vi "Get SMO HELP.vi"(8 "error in (no error)":errorcluster, 10 "Command":string, 11 "Inst.RP100 in":refnum<class "Inst.RP100.lvclass">) -> (0 "error out":errorcluster, 2 "output cluster":T1, 3 "Inst.RP100 out":refnum<class "Inst.RP100.lvclass">)   [LabVIEW 2019, in "Inst.RP100.lvlib" / "Inst.RP100.lvclass"]
uses:
  Inst.RP100.lvclass
  <userlib>/LevyLab/Instrument Framework/subsystems/Help/typedefs/Help--cluster.ctl
  Typedefs/setLevel--Cluster.ctl
  Typedefs/Channel--Num.ctl
  Typedefs/setState--Cluster.ctl
  Typedefs/State--Enum.ctl
  Typedefs/getLevel--Cluster.ctl
  <userlib>/LevyLab/Instrument Framework/Instrument Types/Strain/Instrument.Strain.lvclass
  <vilib>/PRIrvin/JSON-Schema/JSON-Schema.lvlib
  <userlib>/LevyLab/Instrument Framework/subsystems/Help/Help.lvclass
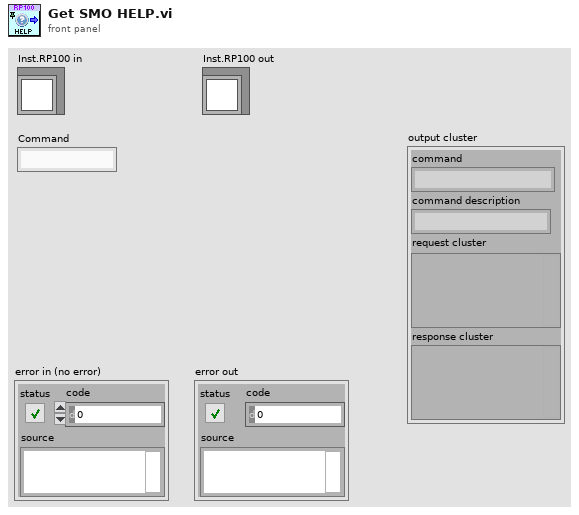
[diagram p1: front panel]
types:
  T1 = typedef "Instrument.lvlib/Help.lvclass/Help--cluster.ctl" = cluster{"command":string, "command description":string, "request cluster":variant, "response cluster":variant}
  T2 = typedef "Inst.RP100.lvlib/Inst.RP100.lvclass/setLevel--Cluster.ctl" = cluster{"channel":T3, "level":dbl, "slew":dbl}
  T3 = typedef "Inst.RP100.lvlib/Inst.RP100.lvclass/Channel--Num.ctl" = i32
  T4 = typedef "Inst.RP100.lvlib/Inst.RP100.lvclass/setState--Cluster.ctl" = cluster{"State":T5}
  T5 = typedef "Inst.RP100.lvlib/Inst.RP100.lvclass/State--Enum.ctl" = enum16{"Shorted", "Enabled"}
  T6 = typedef "Inst.RP100.lvlib/Inst.RP100.lvclass/getLevel--Cluster.ctl" = cluster{"Channel":T3}
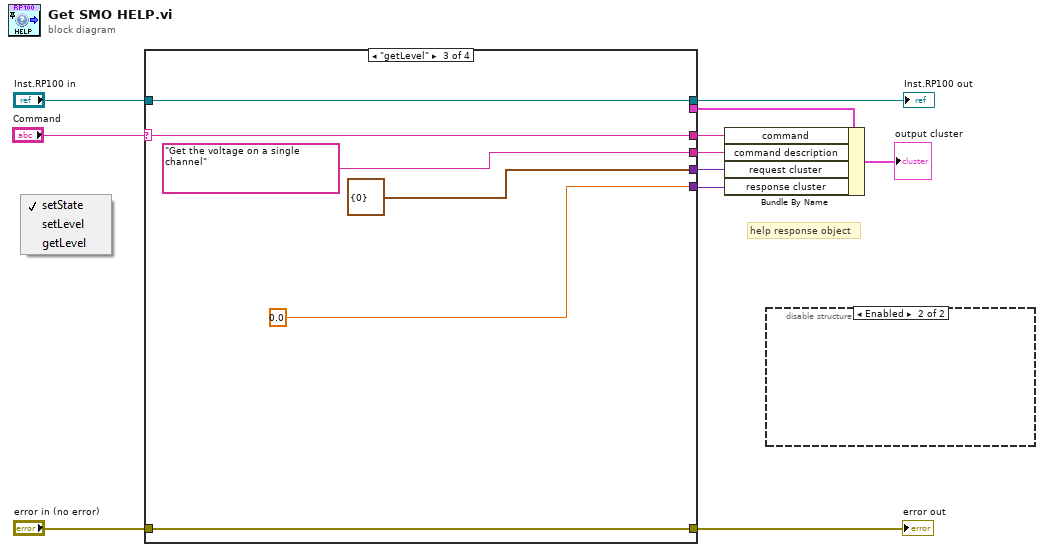
[diagram p0: block diagram]
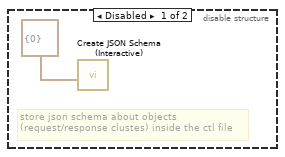
[diagram p2: hidden frame]
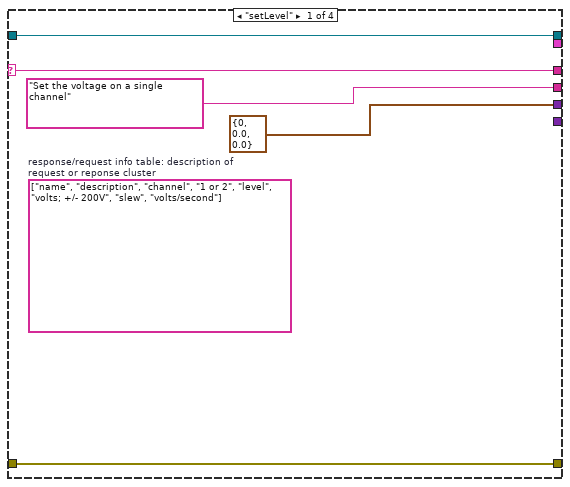
[diagram p3: hidden frame]
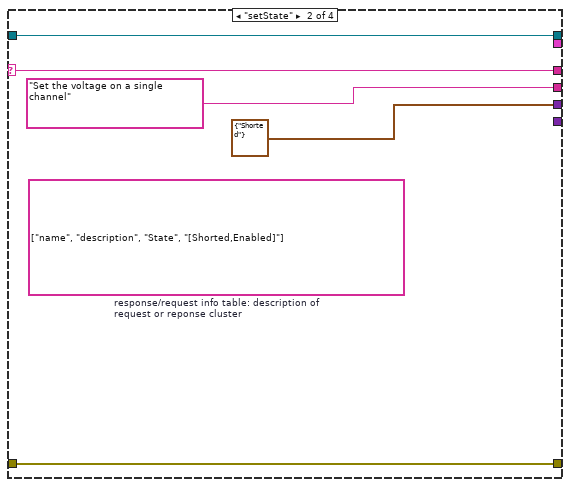
[diagram p4: hidden frame]
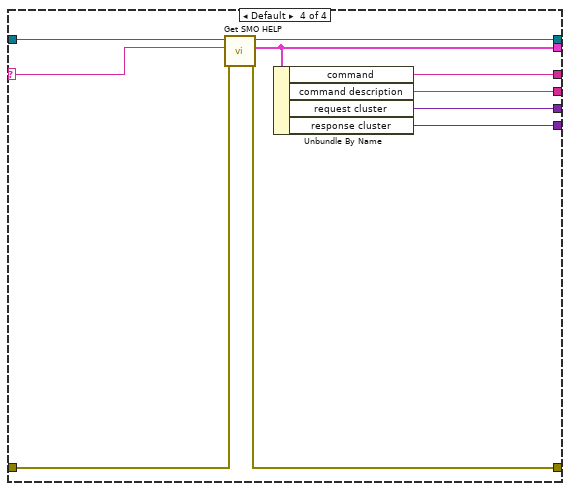
[diagram p5: hidden frame]
diagram:
  # "help response object"
  n1 = case shown="\"getLevel\"" "Command" {
    selector: "Command" -> [w16 w21 w27 w33]
    tunnel: [w16 w21 w27 w31] -> w7
    tunnel: "error in (no error)" -> [w15 w20 w26 w35]
    tunnel: [w15 w20 w26 w34] -> w9
    tunnel: ["Set the voltage on a single channel" "Set the voltage on a single channel" "Get the voltage on a single channel" w30] -> w6
    tunnel: [T2 {"channel"=0, "level"=0.0, "slew"=0.0} ("setLevel") T4 {"State"=enum."Shorted"} ("setState") T6 {"Channel"=0} ("getLevel") w29] -> w5
    tunnel: [_ _ 0.0 ("Level (V)") w28] -> w4
    tunnel: "Inst.RP100 in" -> [w13 w18 w24 w37]
    tunnel: [w13 w18 w24 w36] -> w2
    tunnel: [_ _ _ w32] -> w1
    frame "setLevel" {
      (unwired) string[][] [["name", "description"], ["channel", "1 or 2"], ["level", "volts; +/- 200V"], ["slew", "volts/second"]]  # response/request info table: description of request or reponse cluster
    }
    frame "setState" {
      (unwired) string[][] [["name", "description"], ["State", "[Shorted,Enabled]"]]  # response/request info table: description of request or reponse cluster
    }
    frame "getLevel" {
    }
    frame Default {
      n2 = call-parent "Get SMO HELP.vi"("error in (no error)"=w35, "Command"=w33, "Instrument.Strain in"=w37) -> ("error out"=w34:errorcluster, "help cluster"=w32:T1, "Instrument.Strain out"=w36:refnum<class "Inst.RP100.lvclass">)  [unwired: 6 in]
      n3 = Unbundle By Name(w32) -> ("command"=w31:string, "command description"=w30:string, "request cluster"=w29:variant, "response cluster"=w28:variant)
    }
  }
  "Inst.RP100 out" <- w2
  "error out" <- w9
  n4 = Bundle By Name(cluster=w1, "command"=w7, "command description"=w6, "request cluster"=w5, "response cluster"=w4) -> (→"output cluster":T1)
  n5 = disable-structure shown="Enabled" {
    frame Disabled {
      # "store json schema about objects\n(request/response clustes) inside the ctl file"
      n6 = call <vilib>:"Create JSON Schema (Interactive).vi"("LV Object"=T6 {"Channel"=0} ("getLevel")) -> ()  [unwired: 9 in, 2 out]
    }
    frame Enabled {
    }
  }
